vi "Lookup Table.vi"(11 "Speed":i32) -> (0 "I":dbl, 2 "P":dbl)   [LabVIEW 2016]
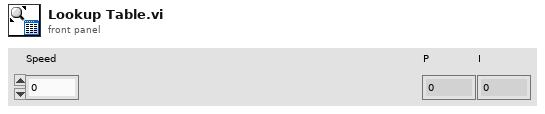
[diagram p1: front panel]
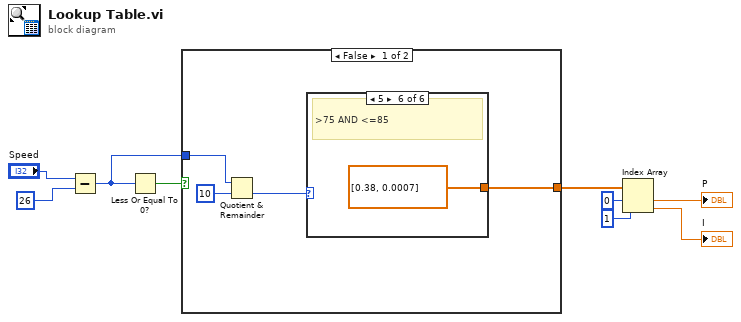
[diagram p0: block diagram]
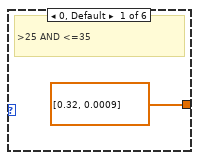
[diagram p2: hidden frame]
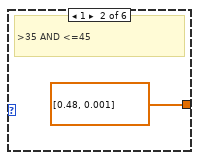
[diagram p3: hidden frame]
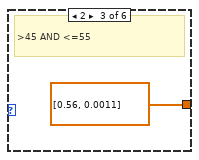
[diagram p4: hidden frame]
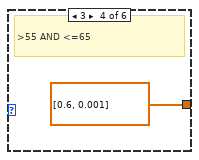
[diagram p5: hidden frame]
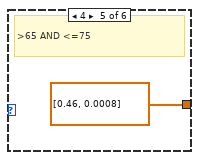
[diagram p6: hidden frame]
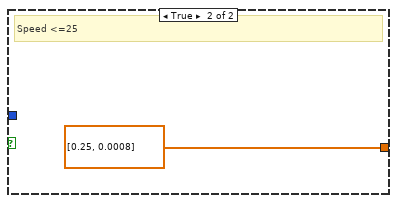
[diagram p7: hidden frame]
diagram:
  n1 = Subtract(x="Speed", y=26) -> (x-y=w6:i32)
  n2 = Less Or Equal To 0?(x=w6) -> (x <= 0?=w7:bool)
  n3 = case shown="False" w7 {
    tunnel: w6 -> [w13 _]
    tunnel: [w10 dbl[] [0.25, 0.0008]] -> w5
    frame False {
      n4 = Quotient & Remainder(x=w13, y=10) -> (floor(x/y)=w11:i32)  [unwired: 1 out]
      n5 = case shown="5" w11 {
        tunnel: [dbl[] [0.32, 0.0009] dbl[] [0.48, 0.001] dbl[] [0.56, 0.0011] dbl[] [0.6, 0.001] dbl[] [0.46, 0.0008] dbl[] [0.38, 0.0007]] -> w10
        frame 0, Default {
          # ">25 AND <=35"
        }
        frame 1 {
          # ">35 AND <=45"
        }
        frame 2 {
          # ">45 AND <=55"
        }
        frame 3 {
          # ">55 AND <=65"
        }
        frame 4 {
          # ">65 AND <=75"
        }
        frame 5 {
          # ">75 AND <=85"
        }
      }
    }
    frame True {
      # "Speed <=25"
    }
  }
  n6 = Index Array(array=w5, index #1=0 ("index"), index #2=1 ("index")) -> (element #1=→"P":dbl, element #2=→"I":dbl)
